vi "Get Config Log.vi"(7 "Default Timestamp":u64, 8 "error in (no error)":errorcluster, 10 "Parse All":bool, 11 "Plugin Manager in":refnum<class "CIFPluginManager.lvclass">) -> (0 "error out":errorcluster, 2 "Filtered Config Entries":string, 3 "Plugin Manager out":refnum<class "CIFPluginManager.lvclass">)   [LabVIEW 2021, in "CIFPluginManager.lvclass"]
uses:
  CIFPluginManager.lvclass
  CIFPluginManager.lvclass/CIFPluginManager.ctl
  CIFUtilities/CIFLogs/CIFLogs.lvlib
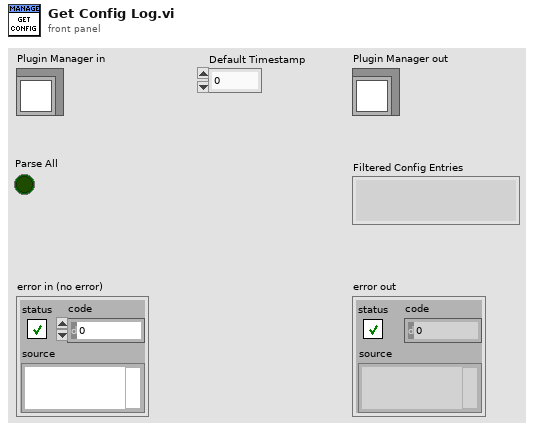
[diagram p1: front panel]
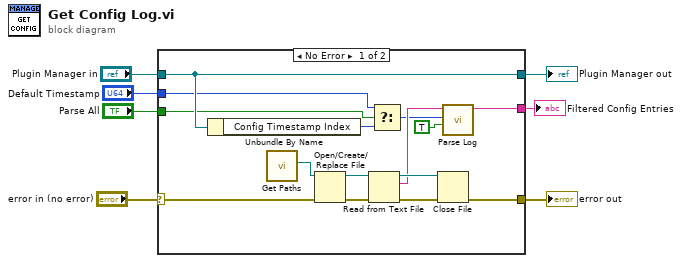
[diagram p0: block diagram]
diagram:
  n1 = case shown="No Error" "error in (no error)" {
    selector: "error in (no error)" -> [w20 w24]
    tunnel: [w17 w24] -> w6
    tunnel: [w16 w23] -> w4
    tunnel: "Plugin Manager in" -> [w16 w23]
    tunnel: [w10 _] -> w2
    tunnel: "Parse All" -> [w14 _]
    tunnel: "Default Timestamp" -> [w8 _]
    frame No Error {
      n2 = Unbundle By Name(w16) -> ("Config Timestamp Index"=w15:u64)
      n3 = call "Get Paths.vi"() -> ("Config Log"=w12:path)  [unwired: 9 in, 2 out]
      n4 = Open/Create/Replace File(file path (use dialog)=w12, error in=w20) -> (refnum out=w21:refnum<file>, error out=w19:errorcluster)  [unwired: 4 in, 1 out]
      n5 = Read from Text File(file (use dialog)=w21, error in=w19) -> (refnum out=w22:refnum<file>, text=w13:string, error out=w18:errorcluster)  [unwired: 2 in, 1 out]
      n6 = Select(t=w8, s=w14, f=w15) -> (s? t:f=w11:u64)
      n7 = Close File(refnum=w22, error in=w18) -> (error out=w17:errorcluster)  [unwired: 1 out]
      n8 = call "Parse Log.vi"("Strip Timestamp"=TRUE, "Index Timestamp"=w11, "Log"=w13) -> ("Filtered Config Entries"=w10:string)  [unwired: 8 in]
    }
    frame Error {
    }
  }
  "error out" <- w6
  "Plugin Manager out" <- w4
  "Filtered Config Entries" <- w2
